vi "QCA Change Channels.vi"(0 "Channel":i32) -> ()   [LabVIEW 2009]
uses:
  QCA Global.vi
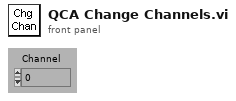
[diagram p1: front panel]
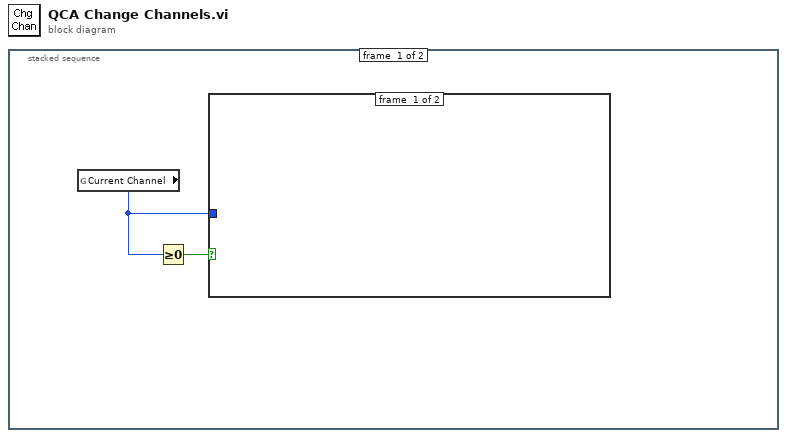
[diagram p0: block diagram]
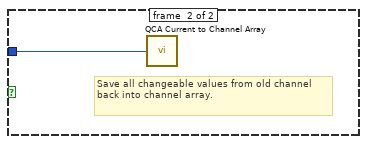
[diagram p2: hidden frame]
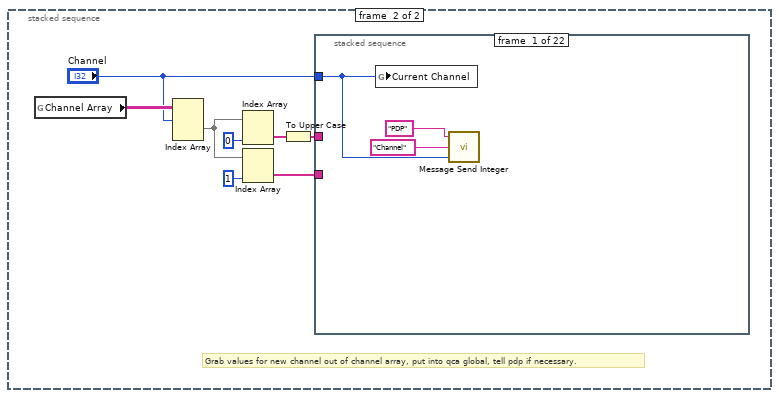
[diagram p3: hidden frame]
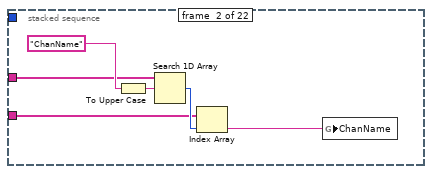
[diagram p4: hidden frame]
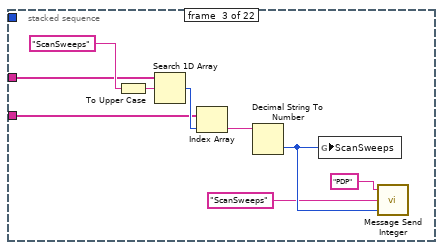
[diagram p5: hidden frame]
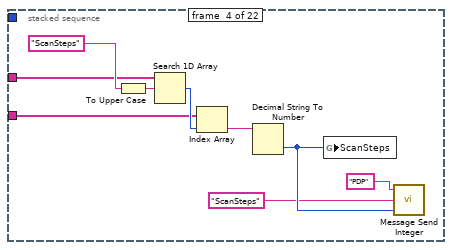
[diagram p6: hidden frame]
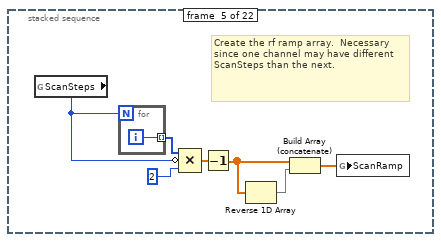
[diagram p7: hidden frame]
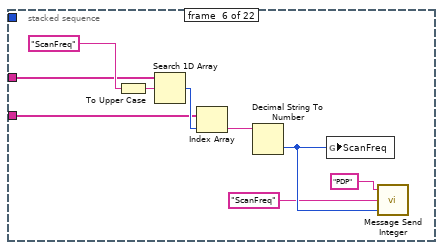
[diagram p8: hidden frame]
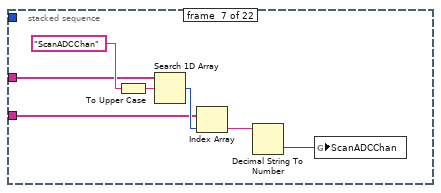
[diagram p9: hidden frame]
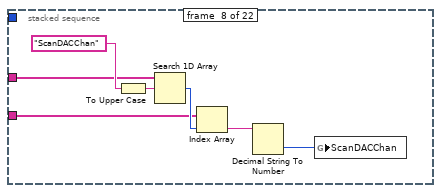
[diagram p10: hidden frame]
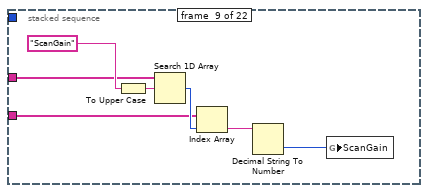
[diagram p11: hidden frame]
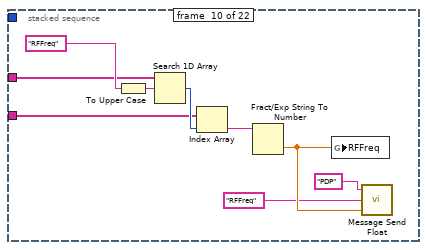
[diagram p12: hidden frame]
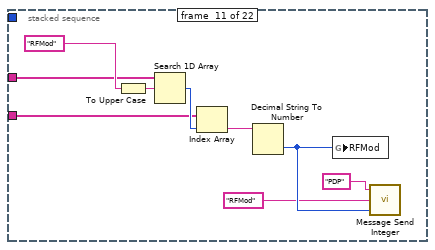
[diagram p13: hidden frame]
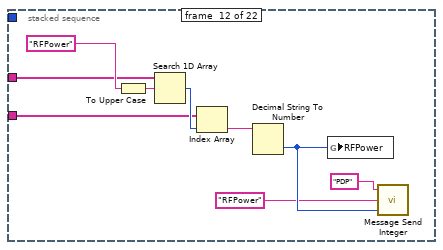
[diagram p14: hidden frame]
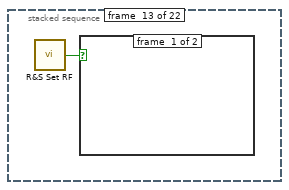
[diagram p15: hidden frame]
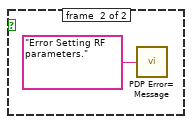
[diagram p16: hidden frame]
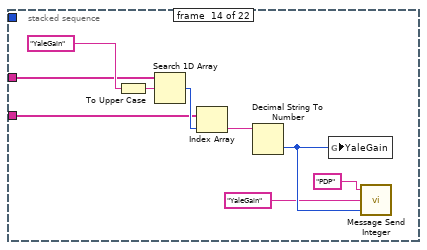
[diagram p17: hidden frame]
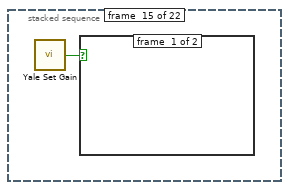
[diagram p18: hidden frame]
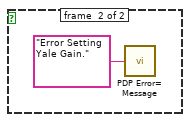
[diagram p19: hidden frame]
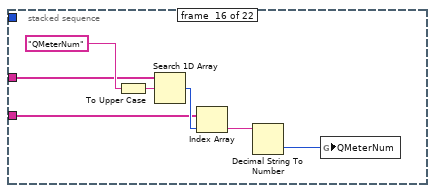
[diagram p20: hidden frame]
diagram:
  n1 = stacked-sequence {
    frame #0 {
      n2 = global read "QCA Global.vi" "Current Channel"() -> (w1:i32)
      n3 = Greater Or Equal To 0?(x=w1) -> (x >= 0?=w2:bool)
      n4 = case shown="True" w2 {
        tunnel: w1 -> [_ w3]
        frame #0 {
        }
        frame #1 {
          # "Save all changeable values from old channel back into channel array."
          n5 = call "QCA Current to Channel Array.vi"("Channel Number"=w3) -> ()
        }
      }
    }
    frame #1 {
      # "Grab values for new channel out of channel array, put into qca global, tell pdp if necessary."
      n6 = global read "QCA Global.vi" "Channel Array"() -> (w10:string[][][])
      n7 = Index Array(array=w10, index (dim 0)="Channel") -> (element=w6:string[][])  [unwired: 2 in]
      n8 = Index Array(array=w6, index (col)=0 ("Index")) -> (element=w9:string[])  [unwired: 1 in]
      n9 = Index Array(array=w6, index (col)=1 ("Index")) -> (element=w7:string[])  [unwired: 1 in]
      n10 = To Upper Case(1:w9) -> (0:w4:string[])
      n11 = stacked-sequence {
        tunnel: w4 -> [_ w17 w26 w35 _ w52 w59 w66 w73 w82 w91 w100 _ w111 _ w120 w128 _ w139 w149 w160 w167]
        tunnel: w7 -> [_ w16 w25 w34 _ w51 w58 w65 w72 w81 w90 w99 _ w110 _ w119 w127 _ w138 w148 w159 w166]
        tunnel: "Channel" -> [w14 _ _ _ _ _ _ _ _ _ _ _ _ _ _ _ _ _ _ _ _ _]
        frame #0 {
          n12 = global write "QCA Global.vi" "Current Channel"(w14) -> ()
          n13 = call "Message Send Integer.vi"("Value"=w14, "Parameter"="Channel", "Destination"="PDP") -> ()
        }
        frame #1 {
          n14 = To Upper Case(1:"ChanName" ("element")) -> (0:w18:string)
          n15 = Search 1D Array(1D array=w17, element=w18) -> (index of element=w19:i32)  [unwired: 1 in]
          n16 = Index Array(array=w16, index=w19) -> (element=w15:string)
          n17 = global write "QCA Global.vi" "ChanName"(w15) -> ()
        }
        frame #2 {
          n18 = To Upper Case(1:"ScanSweeps" ("element")) -> (0:w27:string)
          n19 = Search 1D Array(1D array=w26, element=w27) -> (index of element=w28:i32)  [unwired: 1 in]
          n20 = Index Array(array=w25, index=w28) -> (element=w24:string)
          n21 = Decimal String To Number(string=w24) -> (number=w23:i32)  [unwired: 2 in, 1 out]
          n22 = global write "QCA Global.vi" "ScanSweeps"(w23) -> ()
          n23 = call "Message Send Integer.vi"("Value"=w23, "Parameter"="ScanSweeps", "Destination"="PDP") -> ()
        }
        frame #3 {
          n24 = To Upper Case(1:"ScanSteps" ("element")) -> (0:w36:string)
          n25 = Search 1D Array(1D array=w35, element=w36) -> (index of element=w37:i32)  [unwired: 1 in]
          n26 = Index Array(array=w34, index=w37) -> (element=w33:string)
          n27 = Decimal String To Number(string=w33) -> (number=w32:i32)  [unwired: 2 in, 1 out]
          n28 = global write "QCA Global.vi" "ScanSteps"(w32) -> ()
          n29 = call "Message Send Integer.vi"("Value"=w32, "Parameter"="ScanSteps", "Destination"="PDP") -> ()
        }
        frame #4 {
          # "Create the rf ramp array.  Necessary since one channel may have different ScanSteps than the next."
          n30 = global read "QCA Global.vi" "ScanSteps"() -> (w42:i32)
          n31 = for {
            N: w42 -> [_]
            tunnel: [w46] -> w45 mode=indexing
            i -> [w46]
          }
          n32 = Compound Arithmetic op=MULTIPLY(w45, invert w42, 2 ("Input")) -> (w43:dbl[])
          n33 = Decrement(x=w43) -> (x-1=w40:dbl[])
          n34 = Reverse 1D Array(array=w40) -> (reversed array=w41:dbl[])
          n35 = Build Array (concatenate)(w40, w41) -> (w39:dbl[])
          n36 = global write "QCA Global.vi" "ScanRamp"(w39) -> ()
        }
        frame #5 {
          n37 = To Upper Case(1:"ScanFreq" ("element")) -> (0:w53:string)
          n38 = Search 1D Array(1D array=w52, element=w53) -> (index of element=w54:i32)  [unwired: 1 in]
          n39 = Index Array(array=w51, index=w54) -> (element=w50:string)
          n40 = Decimal String To Number(string=w50) -> (number=w49:i32)  [unwired: 2 in, 1 out]
          n41 = global write "QCA Global.vi" "ScanFreq"(w49) -> ()
          n42 = call "Message Send Integer.vi"("Value"=w49, "Parameter"="ScanFreq", "Destination"="PDP") -> ()
        }
        frame #6 {
          n43 = To Upper Case(1:"ScanADCChan" ("element")) -> (0:w60:string)
          n44 = Search 1D Array(1D array=w59, element=w60) -> (index of element=w61:i32)  [unwired: 1 in]
          n45 = Index Array(array=w58, index=w61) -> (element=w57:string)
          n46 = Decimal String To Number(string=w57) -> (number=w56:i32)  [unwired: 2 in, 1 out]
          n47 = global write "QCA Global.vi" "ScanADCChan"(w56) -> ()
        }
        frame #7 {
          n48 = To Upper Case(1:"ScanDACChan" ("element")) -> (0:w67:string)
          n49 = Search 1D Array(1D array=w66, element=w67) -> (index of element=w68:i32)  [unwired: 1 in]
          n50 = Index Array(array=w65, index=w68) -> (element=w64:string)
          n51 = Decimal String To Number(string=w64) -> (number=w63:i32)  [unwired: 2 in, 1 out]
          n52 = global write "QCA Global.vi" "ScanDACChan"(w63) -> ()
        }
        frame #8 {
          n53 = To Upper Case(1:"ScanGain" ("element")) -> (0:w74:string)
          n54 = Search 1D Array(1D array=w73, element=w74) -> (index of element=w75:i32)  [unwired: 1 in]
          n55 = Index Array(array=w72, index=w75) -> (element=w71:string)
          n56 = Decimal String To Number(string=w71) -> (number=w70:i32)  [unwired: 2 in, 1 out]
          n57 = global write "QCA Global.vi" "ScanGain"(w70) -> ()
        }
        frame #9 {
          n58 = To Upper Case(1:"RFFreq" ("element")) -> (0:w83:string)
          n59 = Search 1D Array(1D array=w82, element=w83) -> (index of element=w84:i32)  [unwired: 1 in]
          n60 = Index Array(array=w81, index=w84) -> (element=w80:string)
          n61 = Fract/Exp String To Number(string=w80) -> (number=w79:dbl)  [unwired: 3 in, 1 out]
          n62 = global write "QCA Global.vi" "RFFreq"(w79) -> ()
          n63 = call "Message Send Float.vi"("Value"=w79, "Parameter"="RFFreq", "Destination"="PDP") -> ()
        }
        frame #10 {
          n64 = To Upper Case(1:"RFMod" ("element")) -> (0:w92:string)
          n65 = Search 1D Array(1D array=w91, element=w92) -> (index of element=w93:i32)  [unwired: 1 in]
          n66 = Index Array(array=w90, index=w93) -> (element=w89:string)
          n67 = Decimal String To Number(string=w89) -> (number=w88:i32)  [unwired: 2 in, 1 out]
          n68 = global write "QCA Global.vi" "RFMod"(w88) -> ()
          n69 = call "Message Send Integer.vi"("Value"=w88, "Parameter"="RFMod", "Destination"="PDP") -> ()
        }
        frame #11 {
          n70 = To Upper Case(1:"RFPower" ("element")) -> (0:w101:string)
          n71 = Search 1D Array(1D array=w100, element=w101) -> (index of element=w102:i32)  [unwired: 1 in]
          n72 = Index Array(array=w99, index=w102) -> (element=w98:string)
          n73 = Decimal String To Number(string=w98) -> (number=w97:i32)  [unwired: 2 in, 1 out]
          n74 = global write "QCA Global.vi" "RFPower"(w97) -> ()
          n75 = call "Message Send Integer.vi"("Value"=w97, "Parameter"="RFPower", "Destination"="PDP") -> ()
        }
        frame #12 {
          n76 = call "R&S Set RF.vi"() -> ("Error"=w104:bool)
          n77 = case shown="True" w104 {
            frame #0 {
            }
            frame #1 {
              n78 = call "PDP Error= Message.vi"("Message"="Error Setting RF parameters.") -> ()
            }
          }
        }
        frame #13 {
          n79 = To Upper Case(1:"YaleGain" ("element")) -> (0:w112:string)
          n80 = Search 1D Array(1D array=w111, element=w112) -> (index of element=w113:i32)  [unwired: 1 in]
          n81 = Index Array(array=w110, index=w113) -> (element=w109:string)
          n82 = Decimal String To Number(string=w109) -> (number=w108:i32)  [unwired: 2 in, 1 out]
          n83 = global write "QCA Global.vi" "YaleGain"(w108) -> ()
          n84 = call "Message Send Integer.vi"("Value"=w108, "Parameter"="YaleGain", "Destination"="PDP") -> ()
        }
        frame #14 {
          n85 = call "Yale Set Gain.vi"() -> ("Error"=w115:bool)
          n86 = case shown="True" w115 {
            frame #0 {
            }
            frame #1 {
              n87 = call "PDP Error= Message.vi"("Message"="Error Setting Yale Gain.") -> ()
            }
          }
        }
        frame #15 {
          n88 = To Upper Case(1:"QMeterNum" ("element")) -> (0:w121:string)
          n89 = Search 1D Array(1D array=w120, element=w121) -> (index of element=w122:i32)  [unwired: 1 in]
          n90 = Index Array(array=w119, index=w122) -> (element=w118:string)
          n91 = Decimal String To Number(string=w118) -> (number=w117:i32)  [unwired: 2 in, 1 out]
          n92 = global write "QCA Global.vi" "QMeterNum"(w117) -> ()
        }
        frame #16 {
          n93 = To Upper Case(1:"QMeterName" ("element")) -> (0:w129:string)
          n94 = Search 1D Array(1D array=w128, element=w129) -> (index of element=w130:i32)  [unwired: 1 in]
          n95 = Index Array(array=w127, index=w130) -> (element=w126:string)
          n96 = global write "QCA Global.vi" "QMeterName"(w126) -> ()
          n97 = call "Message Send Text.vi"("Value"=w126, "Parameter"="QMeterName", "Destination"="PDP") -> ()
        }
        frame #17 {
          n98 = call "QMeter Select.vi"() -> ("Error"=w132:bool)
          n99 = case shown="True" w132 {
            frame #0 {
            }
            frame #1 {
              n100 = call "PDP Error= Message.vi"("Message"="Error Selecting QMeter.") -> ()
            }
          }
        }
        frame #18 {
          n101 = To Upper Case(1:"CalConst" ("element")) -> (0:w140:string)
          n102 = Search 1D Array(1D array=w139, element=w140) -> (index of element=w141:i32)  [unwired: 1 in]
          n103 = Index Array(array=w138, index=w141) -> (element=w137:string)
          n104 = Fract/Exp String To Number(string=w137) -> (number=w136:dbl)  [unwired: 3 in, 1 out]
          n105 = global write "QCA Global.vi" "CalConst"(w136) -> ()
          n106 = call "Message Send Float.vi"("Value"=w136, "Parameter"="CalConst", "Destination"="PDP") -> ()
        }
        frame #19 {
          n107 = To Upper Case(1:"Baseline" ("element")) -> (0:w150:string)
          n108 = Search 1D Array(1D array=w149, element=w150) -> (index of element=w151:i32)  [unwired: 1 in]
          n109 = Index Array(array=w148, index=w151) -> (element=w147:string)
          n110 = Decimal String To Number(string=w147) -> (number=w143:i32)  [unwired: 2 in, 1 out]
          n111 = case shown="1, Default" w143 {
            tunnel: w143 -> [_ _ w156]
            tunnel: ["New Baseline" ("TimeStamp") "No Baseline" ("TimeStamp") w155] -> w146
            frame #0 {
            }
            frame #1 {
            }
            frame #2 {
              n112 = call "Event Number to Timestamp.vi"("Event Number"=w156) -> ("TimeStamp"=w155:string)
            }
          }
          n113 = global write "QCA Global.vi" "Baseline"(w143) -> ()
          n114 = call "Message Send Text.vi"("Value"=w146, "Parameter"="Baseline", "Destination"="PDP") -> ()
        }
        frame #20 {
          n115 = To Upper Case(1:"DCLevelChan" ("element")) -> (0:w161:string)
          n116 = Search 1D Array(1D array=w160, element=w161) -> (index of element=w162:i32)  [unwired: 1 in]
          n117 = Index Array(array=w159, index=w162) -> (element=w158:string)
          n118 = Decimal String To Number(string=w158) -> (number=w157:i32)  [unwired: 2 in, 1 out]
          n119 = global write "QCA Global.vi" "DCLevelChan"(w157) -> ()
        }
        frame #21 {
          n120 = To Upper Case(1:"QMeterTempChan" ("element")) -> (0:w168:string)
          n121 = Search 1D Array(1D array=w167, element=w168) -> (index of element=w169:i32)  [unwired: 1 in]
          n122 = Index Array(array=w166, index=w169) -> (element=w165:string)
          n123 = Decimal String To Number(string=w165) -> (number=w164:i32)  [unwired: 2 in, 1 out]
          n124 = global write "QCA Global.vi" "QMeterTempChan"(w164) -> ()
        }
      }
    }
  }
